vi "Save record.vi"(8 "Error In":errorcluster, 10 "Port":u16=1002, 11 "Address":string="192.168.1.100") -> (0 "Error Out":errorcluster)   [LabVIEW 2015]
panel:
  out "Frame count":i32
  in  "Total samples to read":i32=33554432
  in  "bytes per read":i32=1048576 format="%x"
  in  "Save to File":path=path "D:/Data/dump.bin"
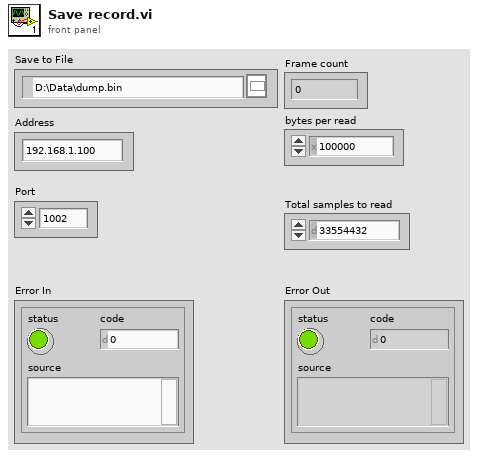
[diagram p1: front panel]
types:
  T1 = enum16{"open", "replace", "create", "open or create", "replace or create", "replace or create with confirmation"}
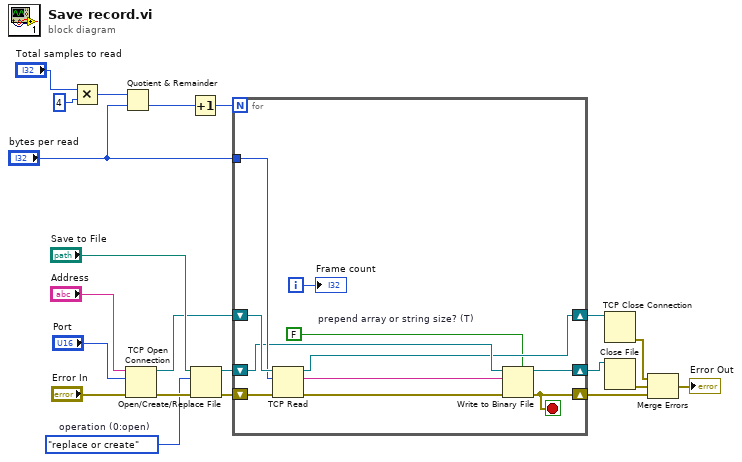
[diagram p0: block diagram]
diagram:
  w16 = T1."replace or create"  # operation (0:open)
  n1 = Multiply(x="Total samples to read", y=4) -> (x*y=w3:i32)
  n2 = Quotient & Remainder(x=w3, y="bytes per read") -> (floor(x/y)=w12:i32)  [unwired: 1 out]
  n3 = TCP Open Connection(address="Address", remote port or service name="Port", error in (no error)="Error In") -> (connection ID=w14:refnum<k5>, error out=w18:errorcluster)  [unwired: 2 in]
  n4 = Increment(x=w12) -> (x+1=w1:i32)
  n5 = Open/Create/Replace File(file path (use dialog)="Save to File", error in=w18, operation (0:open)=w16) -> (refnum out=w10:refnum<file>, error out=w15:errorcluster)  [unwired: 3 in, 1 out]
  n6 = for {
    N: w1 -> [_]
    shift-right: [w24] -> w8
    shift-left: w14 -> [w29]
    shift-right: [w25] -> w5
    shift-left: w15 -> [w32]
    shift-right: [w26] -> w9
    shift-left: w10 -> [w27]
    tunnel: "bytes per read" -> [w28]
    i -> [w23]
    stop <- w25 stop-if-true
    w22 = FALSE  # prepend array or string size? (T)
    n7 = TCP Read(connection ID=w29, bytes to read=w28, error in (no error)=w32) -> (connection ID out=w24:refnum<k5>, data out=w30:string, error out=w31:errorcluster)  [unwired: 2 in]
    n8 = Write to Binary File(file (use dialog)=w27, data=w30, error in=w31, 5:w22) -> (refnum out=w26:refnum<file>, error out=w25:errorcluster)  [unwired: 2 in, 1 out]
    "Frame count" <- w23
  }
  n9 = TCP Close Connection(connection ID=w8) -> (error out=w7:errorcluster)  [unwired: 2 in, 1 out]
  n10 = Close File(refnum=w9) -> (error out=w6:errorcluster)  [unwired: 1 in, 1 out]
  n11 = Merge Errors(w7, w6, w5) -> (→"Error Out":errorcluster)
